vi "Main FPGA.vi"() -> ()   [LabVIEW 2019]
uses:
  <vilib>/rvi/Emulation/niFpgaSctlEmulationGetInTimedLoop.vi
  <vilib>/rvi/Emulation/niFpgaProcessEmulError.vi
  <vilib>/rvi/Emulation/niFpgaGetClockAttributes.vi
  <vilib>/rvi/Emulation/niFpgaEmulationReportErrorSimple.vi
  <vilib>/rvi/Emulation/niFpgaCriticalErrorInLSC.vi
  HD44780/HD44780.lvlib
panel:
  out "Cmd Executed":bool
  out "Display Ready":bool
  out "Data Out":u8 format="%x"
  in  "R/W":bool
  in  "RS":bool
  in  "Data In":u8=12 format="%x"
  in  "Enable":bool
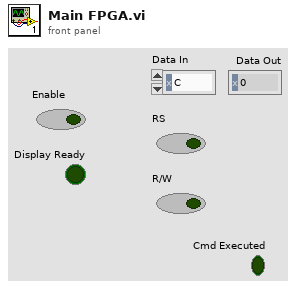
[diagram p1: front panel]
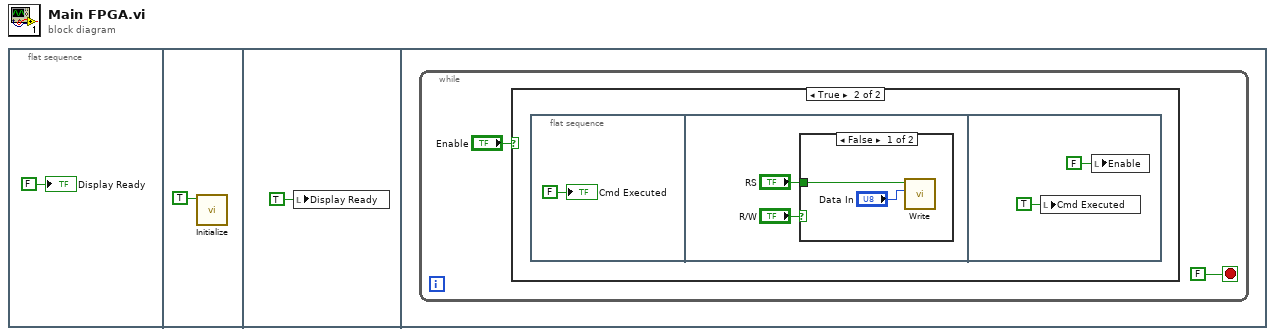
[diagram p0: block diagram]
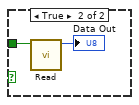
[diagram p3: hidden frame]
diagram:
  n1 = flat-sequence {
    frame #0 {
      "Display Ready" <- FALSE ("Display Ready")
    }
    frame #1 {
      n2 = call "Initialize.vi"("2 Lines?"=TRUE) -> ()  [unwired: 11 in]
    }
    frame #2 {
      n3 = local write "Display Ready"(TRUE ("Display Ready")) -> ()
    }
    frame #3 {
      n4 = while {
        stop <- FALSE stop-if-true
        n5 = case shown="True" "Enable" {
          frame False {
          }
          frame True {
            n6 = flat-sequence {
              frame #0 {
                "Cmd Executed" <- FALSE ("Cmd Executed")
              }
              frame #1 {
                n7 = case shown="False" "R/W" {
                  tunnel: "RS" -> [w10 w12]
                  frame False {
                    n8 = call "Write.vi"("Data"="Data In", "Register Select"=w10) -> ()  [unwired: 10 in]
                  }
                  frame True {
                    n9 = call "Read.vi"("Register Select"=w12) -> ("Data"=→"Data Out":u8)  [unwired: 10 in]
                  }
                }
              }
              frame #2 {
                n10 = local write "Cmd Executed"(TRUE ("Cmd Executed")) -> ()
                n11 = local write "Enable"(FALSE ("Write")) -> ()
              }
            }
          }
        }
      }
    }
  }
